vi "TAT_Select_Varient.vi"(0 "Part List":string[](array[string]), 3 "Error In":errorcluster) -> (7 "User Name Out":string(combo), 8 "Cancle":bool, 9 "Varient no":i32, 10 "error out":errorcluster)   [LabVIEW 2017]
panel:
  in  "Cancel":bool
  in  "OK Button":bool
  in  "Part Name":string(combo)
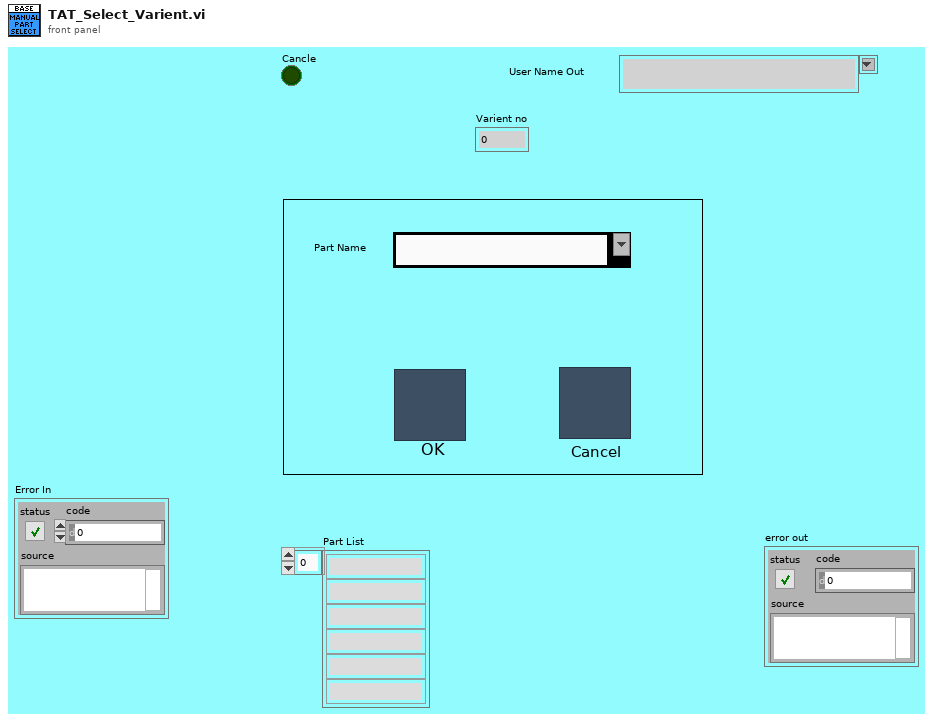
[diagram p1: front panel]
types:
  T1 = enum32{"Invalid", "Standard", "Closed", "Hidden", "Minimized", "Maximized"}
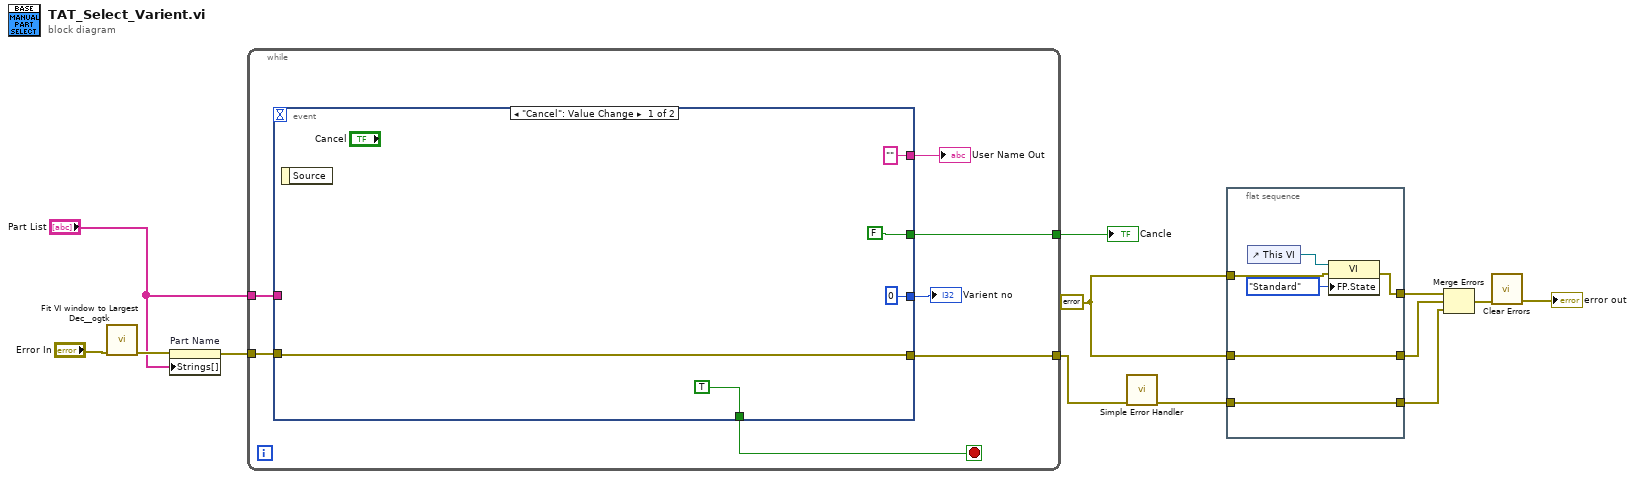
[diagram p0: block diagram]
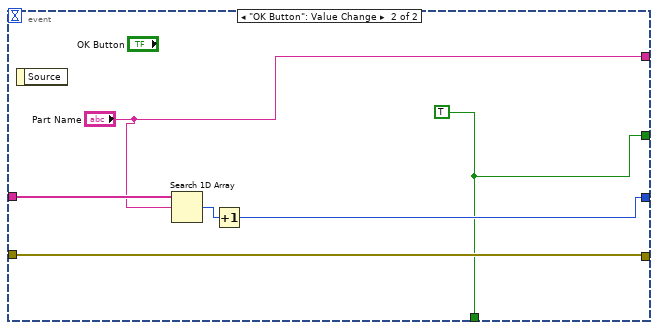
[diagram p2: hidden frame]
diagram:
  w12 = errorcluster {"status"=FALSE, "code"=0, "source"=""} ("error in (no error)")
  n1 = call <userlib>:"Fit VI window to Largest Dec__ogtk.vi"("error in (no error)"="Error In") -> ("error out"=w3:errorcluster)  [unwired: 5 in, 1 out]
  n2 = property on="Part Name" class="CmbBox"(error in=w3, "Strings[]"="Part List") -> (error out=w5:errorcluster)  [unwired: 1 in, 1 out]
  n3 = while {
    tunnel: [w19] -> w13
    tunnel: w5 -> [w18]
    tunnel: [w16] -> w2
    tunnel: "Part List" -> [w15]
    stop <- w20 stop-if-true
    n4 = event shown="[0] \"Cancel\": Value Change" {
      selector: _ -> [_ _]
      dyn-events: _ -> [_ _]
      timeout: _ -> [_ _]
      tunnel: [TRUE w27] -> w20
      tunnel: [w25 w31] -> w19
      tunnel: w18 -> [w25 w31]
      tunnel: [0 ("value") w28] -> w17
      tunnel: [FALSE w27] -> w16
      tunnel: w15 -> [_ w30]
      tunnel: ["" ("Part Name") "Part Name"] -> w14
      event "Cancel": Value Change {
        n5 = event-data() -> ()  [unwired: 1 in, 1 out]
      }
      event "OK Button": Value Change {
        w27 = TRUE
        n6 = event-data() -> ()  [unwired: 1 in, 1 out]
        n7 = Search 1D Array(1D array=w30, element="Part Name") -> (index of element=w29:i32)  [unwired: 1 in]
        n8 = Increment(x=w29) -> (x+1=w28:i32)
      }
    }
    "Varient no" <- w17
    "User Name Out" <- w14
  }
  "Cancle" <- w2
  n9 = call <vilib>:"Simple Error Handler.vi"("error in (no error)"=w13) -> ("error out"=w6:errorcluster)  [unwired: 4 in, 4 out]
  n10 = flat-sequence {
    tunnel: w12 -> [w35]
    tunnel: [w34] -> w11
    tunnel: [w33] -> w8
    tunnel: w12 -> [w33]
    tunnel: [w32] -> w7
    tunnel: w6 -> [w32]
    frame #0 {
      n11 = control-ref of="This VI"() -> (w37:refnum<vi>)
      n12 = property class="VI"(reference=w37, error in=w35, "FP.State"=T1."Standard" ("Front Panel Window:State")) -> (error out=w34:errorcluster)  [unwired: 1 out]
    }
  }
  n13 = Merge Errors(w11, w8, w7) -> (w10:errorcluster)
  n14 = call <vilib>:"Clear Errors.vi"("error in (no error)"=w10) -> ("error out"=→"error out":errorcluster)  [unwired: 5 in, 1 out]
